vi "extractScanMode.vi"(8 "error in (no error)":errorcluster, 11 "Model in":refnum<class "Model.lvclass">) -> (0 "error out":errorcluster, 3 "Model out":refnum<class "Model.lvclass">)   [LabVIEW 2013, in "Model.lvclass"]
uses:
  Model.lvclass
  <userlib>/Common/ILC/ILCModelTypedefs/FinalDelimiter.ctl
  Model.lvclass/Model.ctl
  <userlib>/Common/ILC/Configuration/InputChannels.ctl
  <userlib>/Common/ILC/ILCModelTypedefs/ILCModelTypedefs.lvlib
  <userlib>/Common/ILC/Configuration/ILCConfiguration.lvlib
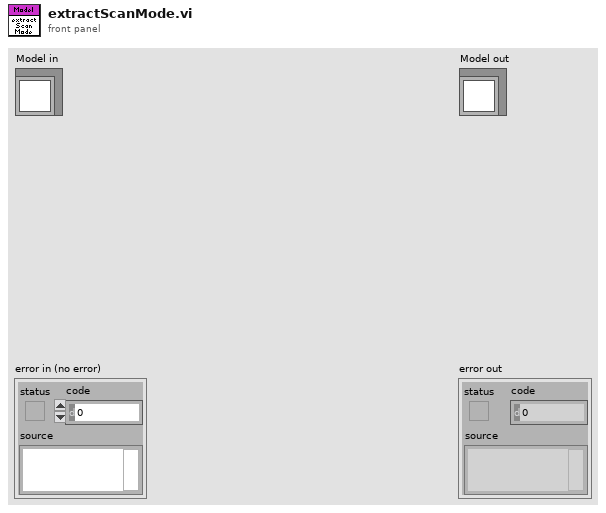
[diagram p1: front panel]
types:
  T1 = typedef "ILCCommon.lvlib/ILCModelTypedefs.lvlib/FinalDelimiter.ctl" = enum16{",", "<CR><LF>"}
  T2 = typedef "ILCCommon.lvlib/ILCConfiguration.lvlib/InputChannels.ctl" = enum16{"Channel 0", "3 Channels", "5 Channels"}
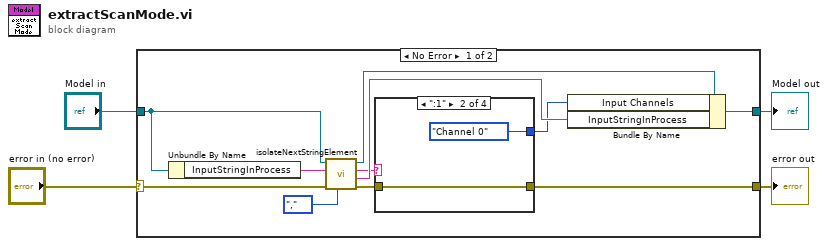
[diagram p0: block diagram]
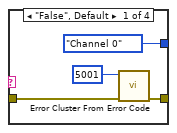
[diagram p2: hidden frame]
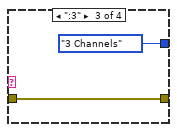
[diagram p3: hidden frame]
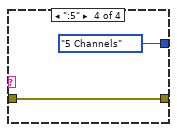
[diagram p4: hidden frame]
diagram:
  n1 = case shown="No Error" "error in (no error)" {
    selector: "error in (no error)" -> [w13 w27]
    tunnel: [w6 w27] -> w3
    tunnel: [w14 w26] -> w1
    tunnel: "Model in" -> [w11 w26]
    frame No Error {
      n2 = Unbundle By Name(w11) -> ("InputStringInProcess"=w12:string)
      n3 = call "isolateNextStringElement.vi"("Final Delimiter"=FinalDelimiter.",", "error in (no error)"=w13, "inputString"=w12, "Model in"=w11) -> ("error out"=w7:errorcluster, "remainingString"=w9:string, "extractedSegment"=w8:string, "Model out"=w10:refnum<class "Model.lvclass">)  [unwired: 4 in]
      n4 = case shown="\":1\"" w8 {
        tunnel: w7 -> [w18 w20 w22 w24]
        tunnel: [w17 w20 w22 w24] -> w6
        tunnel: [InputChannels."Channel 0" ("Input Channels") InputChannels."Channel 0" ("Input Channels") InputChannels."3 Channels" ("Input Channels") InputChannels."5 Channels" ("Input Channels")] -> w5
        frame "False", Default {
          n5 = call <vilib>:"Error Cluster From Error Code.vi"("error in (no error)"=w18, "error code (0)"=5001) -> ("error out"=w17:errorcluster)  [unwired: 7 in]
        }
        frame ":1" {
        }
        frame ":3" {
        }
        frame ":5" {
        }
      }
      n6 = Bundle By Name(cluster=w10, "Input Channels"=w5, "InputStringInProcess"=w9) -> (w14:refnum<class "Model.lvclass">)
    }
    frame Error {
    }
  }
  "error out" <- w3
  "Model out" <- w1
